vi "Charger_IPG Shutdown Delay.vi"(5 "Status Refnum":T1, 6 "error in":errorcluster, 8 "delay (10 s)":dbl[unit]=10.0) -> (0 "error out":errorcluster)   [LabVIEW 2020]
uses:
  Charger_Status Refnum.ctl
  Drivers/Charger Test Set/Charger_Input Control.ctl
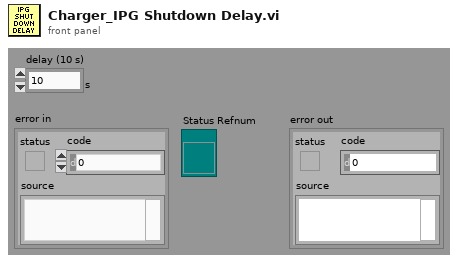
[diagram p1: front panel]
types:
  T1 = typedef "Charger_Status Refnum.ctl" = refnum<vi>
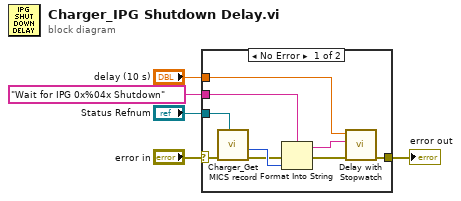
[diagram p0: block diagram]
diagram:
  n1 = case shown="No Error" "error in" {
    selector: "error in" -> [w6 w15]
    tunnel: "Wait for IPG 0x%04x Shutdown" ("window title") -> [w14 _]
    tunnel: "Status Refnum" -> [w13 _]
    tunnel: [w9 w15] -> w3
    tunnel: "delay (10 s)" -> [w7 _]
    frame No Error {
      n2 = call "Charger_Get MICS record.vi"("Status Refnum"=w13, "error in"=w6) -> ("error out"=w11:errorcluster, "ID"=w12:u32)  [unwired: 3 in, 3 out]
      n3 = Format Into String(format string=w14, error in=w11, w12) -> (resulting string=w8:string, error out=w10:errorcluster)  [unwired: 1 in]
      n4 = call "Delay with Stopwatch.vi"("error in"=w10, "window title"=w8, "delay"=w7) -> ("error out"=w9:errorcluster)  [unwired: 4 in]
    }
    frame Error {
    }
  }
  "error out" <- w3
